vi "Write_To_3D_Spreadsheet_w_headers.vi"(0 "Header1":string, 1 "transpose? (no:F)":bool, 2 "format (%.3f)":string="%.3f", 4 "?":path, 5 "append to file? (new file:F)":bool, 6 "1D data":sgl[](array[numeric]) format="%0.2f", 7 "2D data":sgl[][](array[numeric]) format="%0.2f", 8 "3D data":sgl[][][](array[numeric])) -> (3 "new file path (Not A Path if cancelled)":path)   [LabVIEW 2013]
doc: "Converts a 2D or 1D array of single-precision numbers to a text string and writes the string to a new byte stream file or appends the string to an existing file."
panel:
  in  "transpose? (no:F) 2":bool
  in  "format (%.3f) 2":string="%.3f"
  in  "prompt":string="Choose file to write."
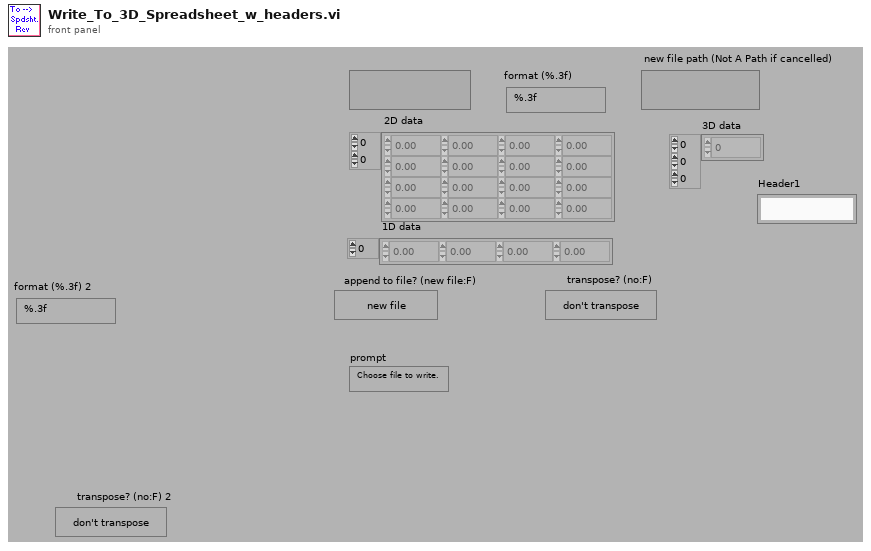
[diagram p1: front panel]
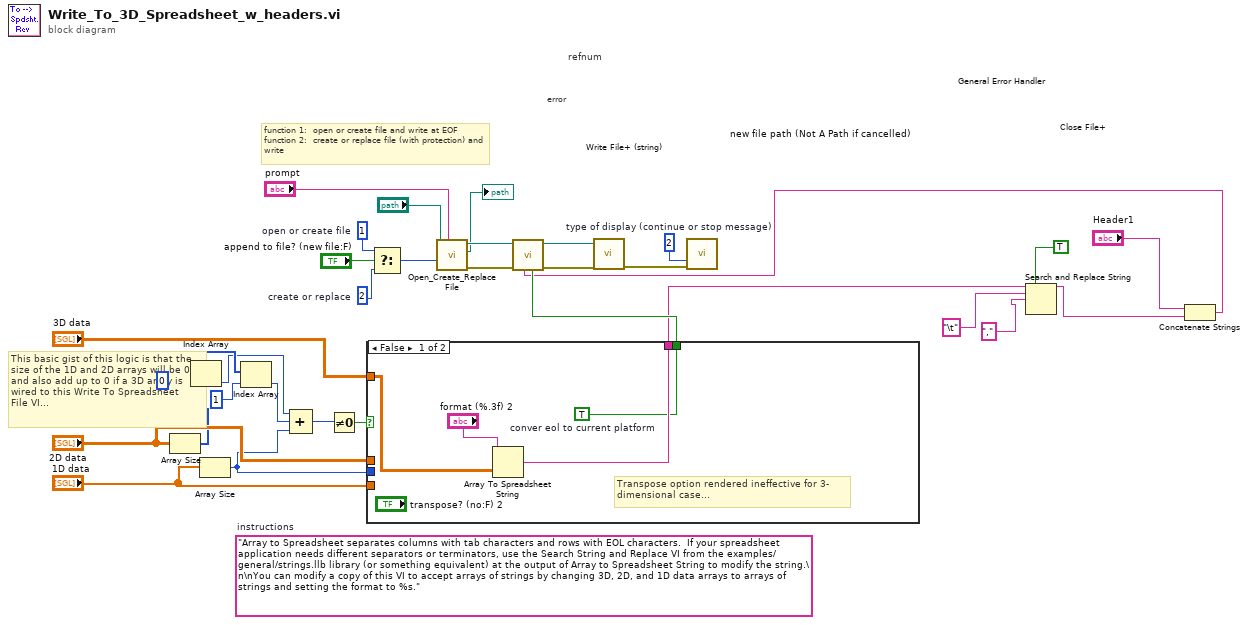
[diagram p0: block diagram]
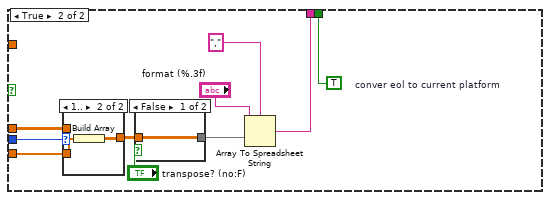
[diagram p2: hidden frame]
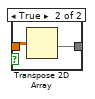
[diagram p3: hidden frame]
diagram:
  (unwired) "Array to Spreadsheet separates columns with tab characters and rows with EOL characters.  If your spreadsheet application needs different separators or terminators, use the Search String and Replace VI from the examples/general/strings.llb library (or something equivalent) at the output of Array to Spreadsheet String to modify the string.\n\nYou can modify a copy of this VI to accept arrays of strings by changing 3D, 2D, and 1D data arrays to arrays of strings and setting the format to %s."  # instructions
  w20 = i16 2  # create or replace
  w30 = 2  # type of display (continue or stop message)
  w31 = i16 1  # open or create file
  # "This basic gist of this logic is that the\nsize of the 1D and 2D arrays will be 0\nand also add up to 0 if a 3D array is\nwired to this Write To Spreadsheet\nFile VI..."
  # "error"
  # "refnum"
  # "function 1:  open or create file and write at EOF\nfunction 2:  create or replace file (with protection) and write"
  n1 = Array Size(array="2D data") -> (size(s)=w15:i32[])
  n2 = Index Array(array=w15, index=0) -> (element=w13:i32)
  n3 = Array Size(array="1D data") -> (size(s)=w11:i32)
  n4 = Index Array(array=w15, index=1) -> (element=w12:i32)
  n5 = Compound Arithmetic op=ADD(w13, w12, w11) -> (w10:i32)
  n6 = Not Equal To 0?(x=w10) -> (x != 0?=w9:bool)
  n7 = case shown="False" w9 {
    tunnel: [w34 w43] -> w4
    tunnel: [w33 w42] -> w23
    tunnel: w11 -> [_ w41]
    tunnel: "1D data" -> [_ w40]
    tunnel: "2D data" -> [_ w39]
    tunnel: "3D data" -> [w35 _]
    frame False {
      w33 = TRUE  # conver eol to current platform
      # "Transpose option rendered ineffective for 3-\ndimensional case..."
      n8 = Array To Spreadsheet String(array=w35, 3:"format (%.3f) 2") -> (spreadsheet string=w34:string)  [unwired: 1 in]
    }
    frame True {
      w42 = TRUE  # conver eol to current platform
      n9 = case shown="1.." w41 {
        tunnel: [w50 w52] -> w45
        tunnel: w40 -> [_ w51]
        tunnel: w39 -> [w50 _]
        frame ..0 {
          # "1D array is empty"
        }
        frame 1.. {
          n10 = Build Array(w51) -> (w52:sgl[][])
        }
      }
      n11 = case shown="False" "transpose? (no:F)" {
        tunnel: [w47 w49] -> w38
        tunnel: w45 -> [w47 w48]
        frame False {
        }
        frame True {
          n12 = Transpose 2D Array(2D array=w48) -> (transposed array=w49:sgl[][])
        }
      }
      n13 = Array To Spreadsheet String(delimiter (Tab)=",", array=w38, 3:"format (%.3f)") -> (spreadsheet string=w43:string)
    }
  }
  n14 = Select(t=w31, s="append to file? (new file:F)", f=w20) -> (s? t:f=w28:i16)
  n15 = call <vilib>:"Open_Create_Replace File.vi"("prompt"="prompt", "function (open:0)"=w28, "file path"="?") -> ("error out"=w26:errorcluster, "new file path"=→"new file path (Not A Path if cancelled)":path, "refnum"=w22:refnum<file>)  [unwired: 5 in, 1 out]
  n16 = Search and Replace String(replace all?=TRUE, input string=w4, search string="\t", replace string=",") -> (result string=w2:string)  [unwired: 4 in, 3 out]
  n17 = Concatenate Strings("Header1", w2) -> (w1:string)
  n18 = call <vilib>:"Write File+ (string).vi"("convert eol? (no:F)"=w23, "string"=w1, "error in (no error)"=w26, "refnum"=w22) -> ("error out"=w29:errorcluster, "dup refnum"=w25:refnum<file>)  [unwired: 3 in, 1 out]
  n19 = call <vilib>:"Close File+.vi"("error in (no error)"=w29, "refnum"=w25) -> ("error out"=w24:errorcluster)  [unwired: 3 in, 2 out]
  n20 = call <vilib>:"General Error Handler.vi"("type of dialog (OK msg:1)"=w30, "error in (no error)"=w24) -> ()  [unwired: 9 in, 5 out]
